vi "GMS Drive.vi"() -> ()   [LabVIEW 2016]
panel:
  in  "Cluster":T1
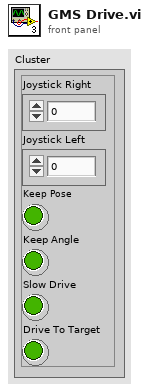
[diagram p1: front panel]
types:
  T1 = cluster{"Joystick Right":dbl, "Joystick Left":dbl, "Keep Pose":bool, "Keep Angle":bool, "Slow Drive":bool, "Drive To Target":bool}
  T2 = typedef "WPI_EncoderDevRef.ctl" = cluster{"DevStatus":errorcluster, "EncoderIndex":T3, "CounterIndex":T4, "DistancePerCount":dbl, "Decoding Type":T5}
  T3 = typedef "FPGA_EncoderIdx.ctl" = enum8{"Enc 0", "Enc 1", "Enc 2", "Enc 3", "Enc 4", "Enc 5", "Enc 6", "Enc 7", "Invalid"}
  T4 = typedef "FPGA_CounterCtrSystemIndex.ctl" = enum8{"Ctr 0", "Ctr 1", "Ctr 2", "Ctr 3", "Ctr 4", "Ctr 5", "Ctr 6", "Ctr 7", "Invalid"}
  T5 = typedef "WPI_EncoderType.ctl" = enum16{"1x", "2x", "4x"}
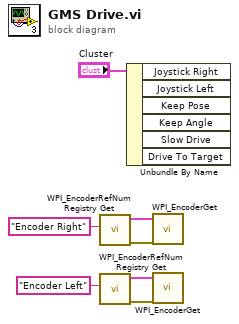
[diagram p0: block diagram]
diagram:
  n1 = call <vilib>:"WPI_EncoderRefNum Registry Get.vi"("refnum name"="Encoder Right") -> ("error out"=w6:errorcluster, "EncoderDevRef"=w5:T2)  [unwired: 9 in]
  n2 = call <vilib>:"WPI_EncoderRefNum Registry Get.vi"("refnum name"="Encoder Left") -> ("error out"=w3:errorcluster, "EncoderDevRef"=w2:T2)  [unwired: 9 in]
  n3 = Unbundle By Name("Cluster") -> ()  [unwired: 6 out]
  n4 = call <vilib>:"WPI_EncoderGet.vi"("error in (no error)"=w6, "EncoderDevRef"=w5) -> ()  [unwired: 4 in, 6 out]
  n5 = call <vilib>:"WPI_EncoderGet.vi"("error in (no error)"=w3, "EncoderDevRef"=w2) -> ()  [unwired: 4 in, 6 out]
